vi "XYGraphTableGen.vi"(0 "NouvDonnées X":dbl, 1 "XData":dbl[](array[numeric]) caption="Tous les DonnX", 2 "TracerCourbe":bool[](array[boolean]), 5 "All XYGraph In":T1(array[cluster]), 7 "NouvDonnées Y":dbl[](array[numeric]), 9 "Actual Point Index":i32, 11 "error in (no error)":errorcluster, 12 "All YData":dbl[][](array[numeric]), 13 "Actual Curve Index":i32) -> (3 "XData Out":dbl[](array[numeric]) caption="Tous les DonnX Out", 6 "All XYGraph Out":T1(array[cluster]), 8 "XYGraph":T1(array[cluster]), 14 "All YData out":dbl[][](array[numeric]), 15 "error out":errorcluster)   [LabVIEW 2010]
doc: "Ce Vi ajoute les nouvelles données acquisitionner dans les tables de toutes les données acquisitionner. Il formate ensuite les données sous forme de cluster pour l'affichage dans un graphique XY."
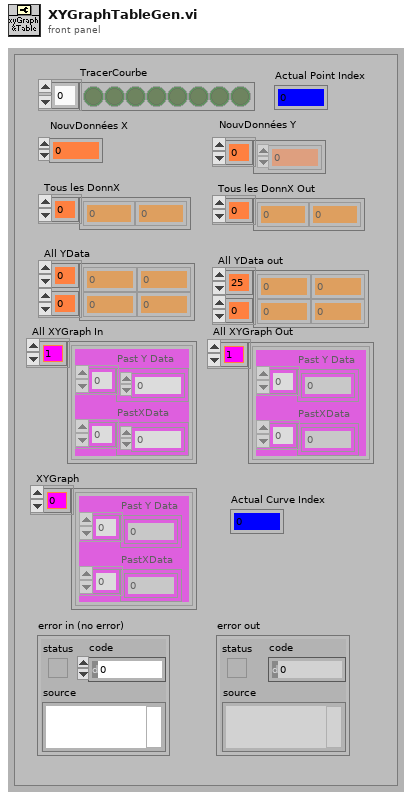
[diagram p1: front panel]
types:
  T1 = cluster{"Past Y Data":dbl[], "PastXData":dbl[]}[]
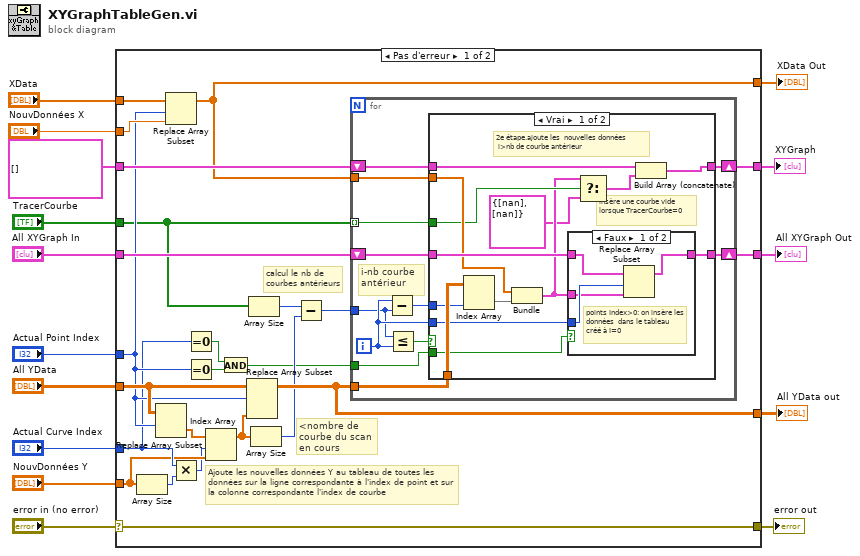
[diagram p0: block diagram]
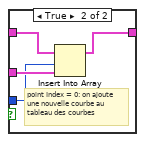
[diagram p2: hidden frame]
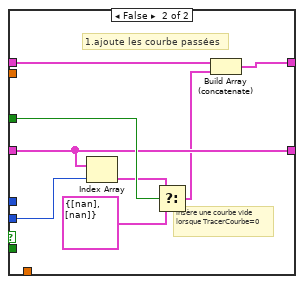
[diagram p3: hidden frame]
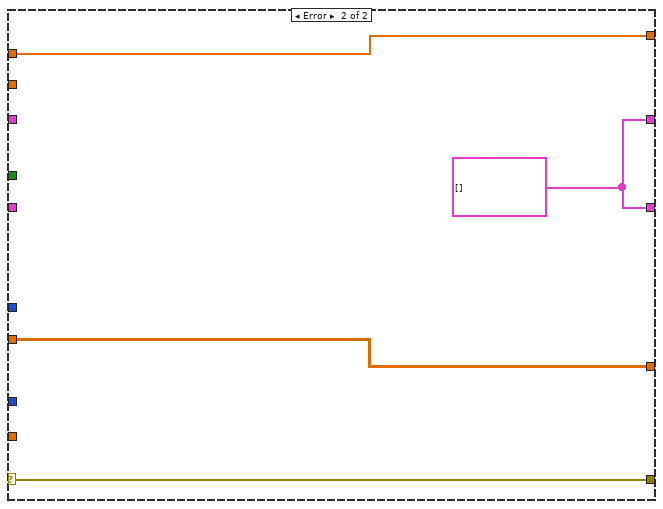
[diagram p4: hidden frame]
diagram:
  n1 = case shown="Pas d'erreur" "error in (no error)" {
    selector: "error in (no error)" -> [w37 w85]
    tunnel: "NouvDonnées Y" -> [w18 _]
    tunnel: "XData" -> [w35 w83]
    tunnel: "NouvDonnées X" -> [w34 _]
    tunnel: "Actual Point Index" -> [w27 _]
    tunnel: "All YData" -> [w28 w84]
    tunnel: [w39 w82] -> w3
    tunnel: [w37 w85] -> w11
    tunnel: [w30 w84] -> w10
    tunnel: [w36 w83] -> w9
    tunnel: "TracerCourbe" -> [w23 _]
    tunnel: T1 [] ("XYGraph In") -> [w38 _]
    tunnel: "All XYGraph In" -> [w32 _]
    tunnel: [w33 w82] -> w2
    tunnel: "Actual Curve Index" -> [w19 _]
    frame No Error {
      # "<nombre de courbe du scan en cours"
      # "calcul le nb de courbes antérieurs"
      # "Ajoute les nouvelles données Y au tableau de toutes les données sur la ligne correspondante à l'index de point et sur la colonne correspondante l'index de courbe"
      n2 = Array Size(array=w18) -> (size(s)=w16:i32)
      n3 = Index Array(array=w28, index (row)=w27) -> (element=w26:dbl[])  [unwired: 1 in]
      n4 = Replace Array Subset(array=w35, new element=w34, index=w27) -> (w36:dbl[])
      n5 = Multiply(x=w19, y=w16) -> (x*y=w17:i32)
      n6 = Equal To 0?(x=w19) -> (x = 0?=w22:bool)
      n7 = Equal To 0?(x=w27) -> (x = 0?=w21:bool)
      n8 = Replace Array Subset(array=w26, new element=w18, index=w17) -> (w25:dbl[])
      n9 = And(x=w22, y=w21) -> (x .and. y?=w20:bool)
      n10 = Replace Array Subset(array=w28, new element=w25, index (row)=w27) -> (w30:dbl[][])  [unwired: 1 in]
      n11 = Array Size(array=w23) -> (size(s)=w24:i32)
      n12 = Array Size(array=w25) -> (size(s)=w29:i32)
      n13 = Subtract(x=w24, y=w29) -> (x-y=w31:i32)
      n14 = for {
        tunnel: w36 -> [w51]
        tunnel: w23 -> [w49] mode=indexing
        shift-right: [w50] -> w39
        shift-left: w38 -> [w48]
        tunnel: w30 -> [w45]
        tunnel: w31 -> [w42]
        shift-right: [w46] -> w33
        shift-left: w32 -> [w41]
        tunnel: w20 -> [w40]
        i -> [w43]
        # "i-nb courbe\nantérieur"
        n15 = Subtract(x=w43, y=w42) -> (x-y=w44:i32)
        n16 = Less Or Equal?(x=w42, y=w43) -> (x <= y?=w47:bool)
        n17 = case shown="Vrai" w47 {
          tunnel: w51 -> [w58 _]
          tunnel: [w61 w77] -> w50
          tunnel: w49 -> [w57 w81]
          tunnel: w48 -> [w62 w78]
          tunnel: w44 -> [w63 _]
          tunnel: [w55 w79] -> w46
          tunnel: w45 -> [w65 _]
          tunnel: w43 -> [w54 w80]
          tunnel: w41 -> [w59 w79]
          tunnel: w40 -> [w53 _]
          frame True {
            # "insère une courbe vide lorsque TracerCourbe=0"
            # "2e étape.ajoute les  nouvelles données\n i>nb de courbe antérieur"
            n18 = Index Array(array=w65, index (col)=w63) -> (element=w64:dbl[])  [unwired: 1 in]
            n19 = Bundle("XData"=w58, "All YData"=w64) -> (w56:cluster{"XData":dbl[], "All YData":dbl[]})  [unwired: 1 in]
            n20 = case shown="Faux" w53 {
              tunnel: w59 -> [w67 w73]
              tunnel: w56 -> [w68 w72]
              tunnel: [w66 w71] -> w55
              tunnel: w54 -> [w69 w70]
              frame False {
                # "points Index>0: on insère les données  dans le tableau créé à I=0"
                n21 = Replace Array Subset(array=w67, new element=w68, index=w69) -> (w66:T1)
              }
              frame True {
                # "point Index = 0: on ajoute une nouvelle courbe au tableau des courbes"
                n22 = Insert Into Array(array=w73, index=w70, new element=w72) -> (w71:T1)
              }
            }
            n23 = Select(t=w56, s=w57, f=cluster{"Past Y Data":dbl[], "PastXData":dbl[]} {"Past Y Data"=[nan], "PastXData"=[nan]}) -> (s? t:f=w60:cluster{"Past Y Data":dbl[], "PastXData":dbl[]})
            n24 = Build Array (concatenate)(w62, w60) -> (w61:T1)
          }
          frame False {
            # "insère une courbe vide lorsque TracerCourbe=0"
            # "1.ajoute les courbe passées"
            n25 = Index Array(array=w79, index=w80) -> (element=w76:cluster{"Past Y Data":dbl[], "PastXData":dbl[]})
            n26 = Select(t=w76, s=w81, f=cluster{"Past Y Data":dbl[], "PastXData":dbl[]} {"Past Y Data"=[nan], "PastXData"=[nan]}) -> (s? t:f=w74:cluster{"Past Y Data":dbl[], "PastXData":dbl[]})
            n27 = Build Array (concatenate)(w78, w74) -> (w77:T1)
          }
        }
      }
    }
    frame Error {
      w82 = cluster{"XData":dbl[], "All YData":dbl[]}[] []
    }
  }
  "error out" <- w11
  "All YData out" <- w10
  "XData Out" <- w9
  "XYGraph" <- w3
  "All XYGraph Out" <- w2
